vi "Get Actor.vi"(11 "Alarming Strategy in":refnum<class "Alarming Actor Strategy.lvclass">) -> (2 "Actor":refnum<class "Actor.lvclass">, 3 "Alarming Strategy out":refnum<class "Alarming Actor Strategy.lvclass">)   [LabVIEW 2024, in "Alarming Actor Strategy.lvclass"]
uses:
  Alarming Actor Strategy.lvclass
  <vilib>/ActorFramework/Actor/Actor.lvclass
  Alarming Actor Strategy.lvclass/Alarming Actor Strategy.ctl
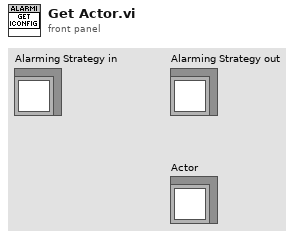
[diagram p1: front panel]
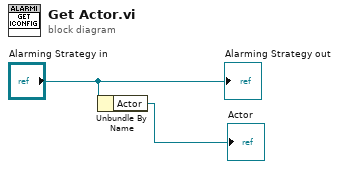
[diagram p0: block diagram]
diagram:
  n1 = Unbundle By Name("Alarming Strategy in") -> ("Actor"=→"Actor":refnum<class "Actor.lvclass">)
  "Alarming Strategy out" <- "Alarming Strategy in"
